vi "svx_Oct_Waterfall Execute.vi"(0 "Data In":T3 {"Plots"."Y" format="%.2f"; "Plots"."X" format="%.2f"}, 1 "Display State In":T2={"X Scale Width %"=80.0, "Y Scale Height %"=40.0, "X-Axis Range"={"Minimum"=0.0, "Maximum"=10.0}, "Y-Axis Range"={"Minimum"=0.0, "Maximum"=10.0}, "Z-Axis Range"={"Minimum"=0.0, "Maximum"=10.0}, "Plot Color"=0, "Frame Color"=61212, "Background Color"=16252785, "Initial AutoScale Y"=TRUE, "AutoScale X"=2, "AutoScale Y"=2, "AutoScale Z"=2, "Plot Transparency"=FALSE, "X-Axis Name"="Frequency", "Y-Axis Name"="Amplitude", "Z-Axis Name"="", "X-Axis Scaling Factor"={"Offset"=0.0, "Multiplier"=1.0}, "Y-Axis Scaling Factor"={"Offset"=0.0, "Multiplier"=1.0}, "Z-Axis Scaling Factor"={"Offset"=0.0, "Multiplier"=1.0}, "X-Scale Visible"=TRUE, "Y-Scale Visible"=TRUE, "Z-Scale Visible"=TRUE, "X-Scale Label Visible"=TRUE, "Y-Scale Label Visible"=TRUE, "Z-Scale Label Visible"=TRUE, "X-Axis Range Scaled"={"Minimum"=0.0, "Maximum"=10.0}, "Y-Axis Range Scaled"={"Minimum"=0.0, "Maximum"=10.0}, "Z-Axis Range Scaled"={"Minimum"=0.0, "Maximum"=10.0}, "Rev Z Order"=FALSE, "X-Scale Format Str"="%#.4g", "Y-Scale Format Str"="%#.4g", "Z-Scale Format Str"="%#.4g", "Decor color"=12369084, "Scale Range Change"=refnum, "out of state queue"=refnum, "property nodes"=refnum} caption="State In", 2 "Container State":T5, 3 "# Plots Updated":i32, 4 "Dec/Cropped in":T3 {"Plots"."Y" format="%.2f"; "Plots"."X" format="%.2f"}, 6 "Execution Tasks":T4[](array[typedef]), 7 "Main Graph":refnum<vi>, 8 "Coords":T1, 9 "XY Scale Graph ref":refnum<vi>, 11 "Z Scale Graph ref":refnum<vi>, 12 "This VI":refnum<vi>, 13 "Background ref":refnum<vi>) -> (14 "Data Out":T3={"z0"=0.0, "dz"=1.0, "Plots"=[]} {"Plots"."Y" format="%.2f"; "Plots"."X" format="%.2f"}, 15 "Display State Out":T2={"X Scale Width %"=80.0, "Y Scale Height %"=40.0, "X-Axis Range"={"Minimum"=0.0, "Maximum"=10.0}, "Y-Axis Range"={"Minimum"=0.0, "Maximum"=10.0}, "Z-Axis Range"={"Minimum"=0.0, "Maximum"=10.0}, "Plot Color"=61212, "Frame Color"=16252785, "Background Color"=16777222, "Initial AutoScale Y"=TRUE, "AutoScale X"=2, "AutoScale Y"=2, "AutoScale Z"=2, "Plot Transparency"=FALSE, "X-Axis Name"="Frequency", "Y-Axis Name"="Amplitude", "Z-Axis Name"="", "X-Axis Scaling Factor"={"Offset"=0.0, "Multiplier"=1.0}, "Y-Axis Scaling Factor"={"Offset"=0.0, "Multiplier"=1.0}, "Z-Axis Scaling Factor"={"Offset"=0.0, "Multiplier"=1.0}, "X-Scale Visible"=TRUE, "Y-Scale Visible"=TRUE, "Z-Scale Visible"=TRUE, "X-Scale Label Visible"=TRUE, "Y-Scale Label Visible"=TRUE, "Z-Scale Label Visible"=TRUE, "X-Axis Range Scaled"={"Minimum"=0.0, "Maximum"=10.0}, "Y-Axis Range Scaled"={"Minimum"=0.0, "Maximum"=10.0}, "Z-Axis Range Scaled"={"Minimum"=0.0, "Maximum"=10.0}, "Rev Z Order"=FALSE, "X-Scale Format Str"="%#.4g", "Y-Scale Format Str"="%#.4g", "Z-Scale Format Str"="%#.4g", "Decor color"=12369084, "Scale Range Change"=refnum, "out of state queue"=refnum, "property nodes"=refnum} caption="State", 17 "# Plots Updated out":i32, 18 "Dec/Cropped out":T3={"z0"=0.0, "dz"=1.0, "Plots"=[]} {"Plots"."Y" format="%.2f"; "Plots"."X" format="%.2f"})   [LabVIEW 2017, in "SVX Octave Waterfall Graph.xctl"]
uses:
  <vilib>/addons/_XControls/Octave Waterfall Graph/SVX Octave Waterfall Graph.xctl
  <vilib>/_xctls/Container State.ctl
  <vilib>/addons/_XControls/Octave Waterfall Graph/subVIs/svx_Oct_Waterfall Data.ctl
  <vilib>/addons/_XControls/Octave Waterfall Graph/subVIs/svx_Oct_Waterfall State.ctl
  <vilib>/addons/_XControls/Octave Waterfall Graph/subVIs/svx_Oct_Waterfall Execution Tasks.ctl
  <vilib>/Utility/miscctls.llb/LVPoint32TypeDef.ctl
  <vilib>/_xctls/XControlSupport.lvlib
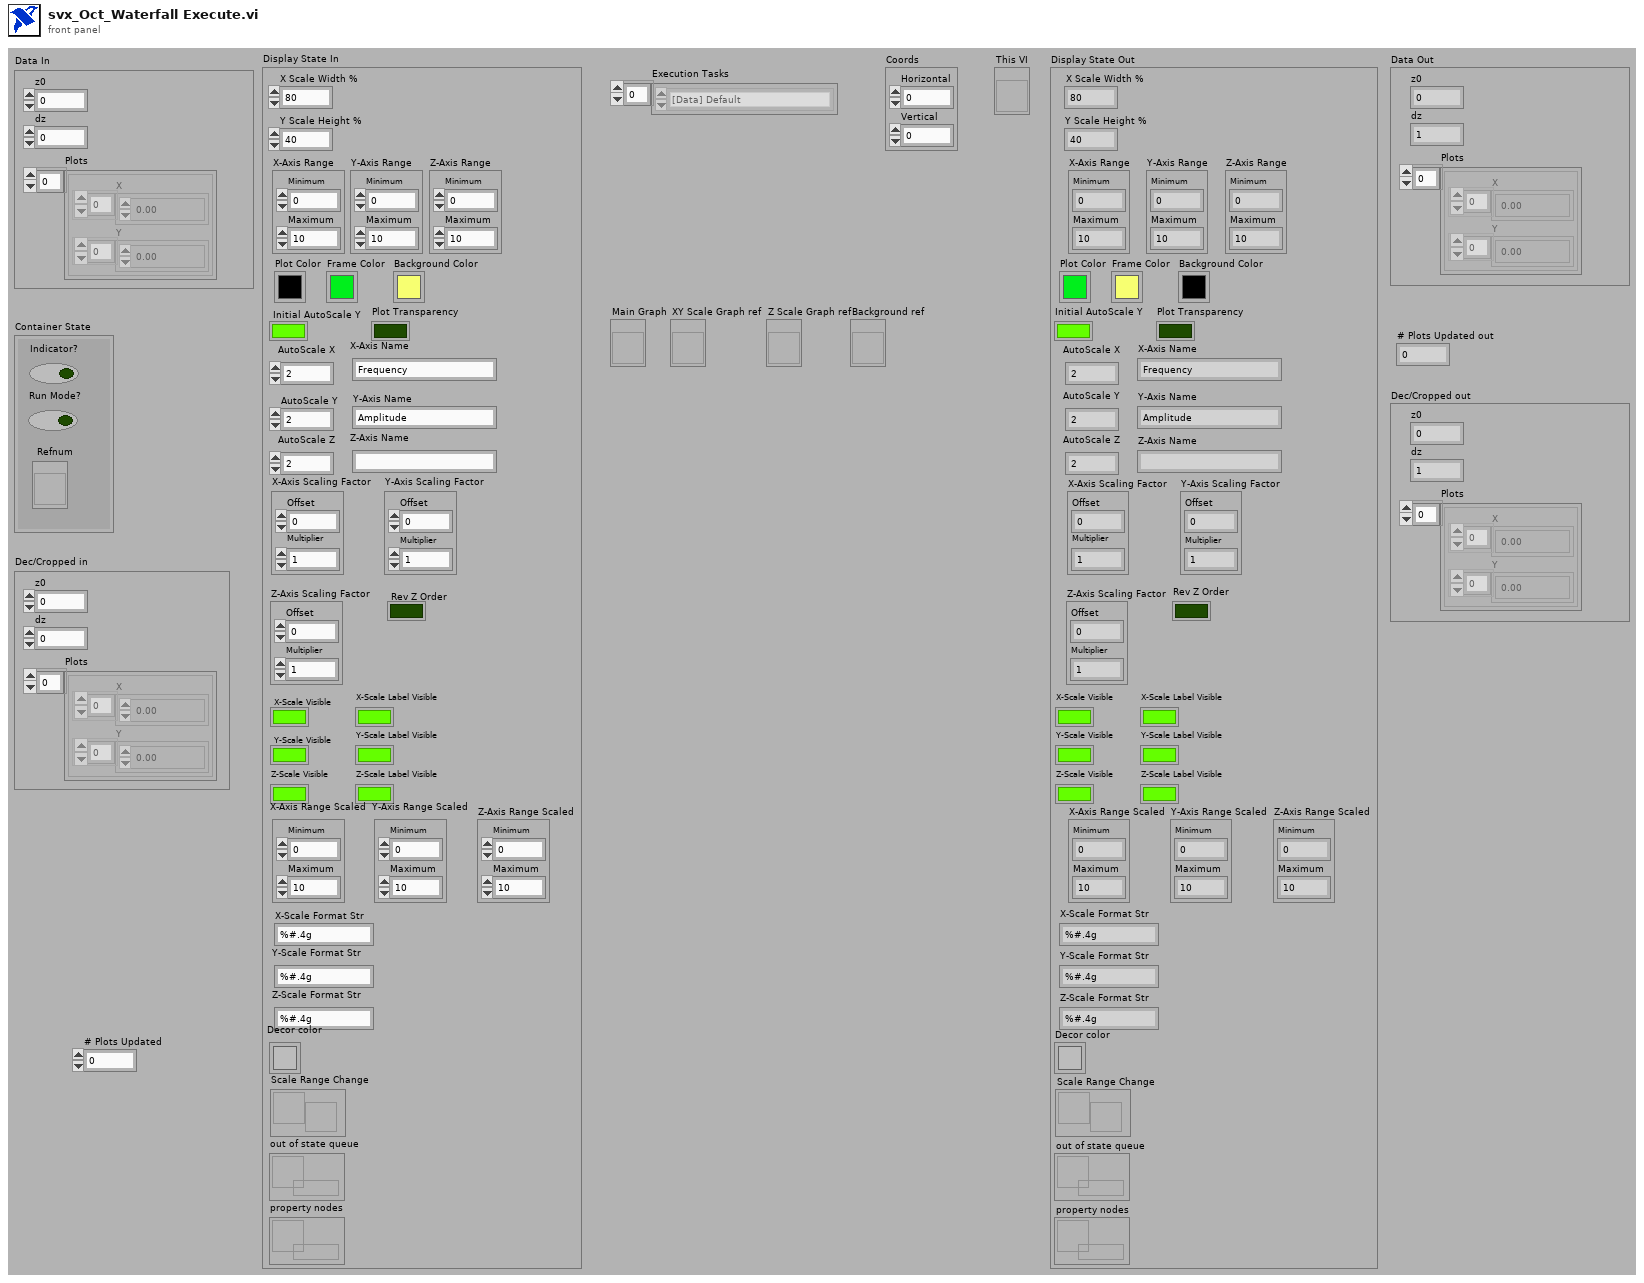
[diagram p1: front panel]
types:
  T1 = typedef "LVPoint32TypeDef.ctl" = cluster{"Horizontal":i32, "Vertical":i32}
  T2 = typedef "SVX Octave Waterfall Graph.xctl/svx_Oct_Waterfall State.ctl" = cluster{"X Scale Width %":dbl, "Y Scale Height %":dbl, "X-Axis Range":cluster{"Minimum":dbl, "Maximum":dbl}, "Y-Axis Range":cluster{"Minimum":dbl, "Maximum":dbl}, "Z-Axis Range":cluster{"Minimum":dbl, "Maximum":dbl}, "Plot Color":u32, "Frame Color":u32, "Background Color":u32, "Initial AutoScale Y":bool, "AutoScale X":u8, "AutoScale Y":u8, "AutoScale Z":u8, "Plot Transparency":bool, "X-Axis Name":string, "Y-Axis Name":string, "Z-Axis Name":string, "X-Axis Scaling Factor":cluster{"Offset":dbl, "Multiplier":dbl}, "Y-Axis Scaling Factor":cluster{"Offset":dbl, "Multiplier":dbl}, "Z-Axis Scaling Factor":cluster{"Offset":dbl, "Multiplier":dbl}, "X-Scale Visible":bool, "Y-Scale Visible":bool, "Z-Scale Visible":bool, "X-Scale Label Visible":bool, "Y-Scale Label Visible":bool, "Z-Scale Label Visible":bool, "X-Axis Range Scaled":cluster{"Minimum":dbl, "Maximum":dbl}, "Y-Axis Range Scaled":cluster{"Minimum":dbl, "Maximum":dbl}, "Z-Axis Range Scaled":cluster{"Minimum":dbl, "Maximum":dbl}, "Rev Z Order":bool, "X-Scale Format Str":string, "Y-Scale Format Str":string, "Z-Scale Format Str":string, "Decor color":u32, "Scale Range Change":refnum<user-event>, "out of state queue":refnum<queue>, "property nodes":refnum<queue>}
  T3 = typedef "SVX Octave Waterfall Graph.xctl/svx_Oct_Waterfall Data.ctl" = cluster{"z0":dbl, "dz":dbl, "Plots":cluster{"X":dbl[], "Y":dbl[]}[]}
  T4 = typedef "SVX Octave Waterfall Graph.xctl/svx_Oct_Waterfall Execution Tasks.ctl" = enum16{"[Data] Default", "[Data] Update Graph", "[Pane] Calculate Size from Coord Change", "[Pane] Calculate Size from Display State", "[Plot] Redraw Frame", "[Plot] Update Plot Color", "[Scale] Autoscale or Crop X, Y, Z", "[Scale] Resize Scales", "[Scale] Align Scale Labels", "[Plot] Initialize Plot", "[Scale] X Scale", "[Scale] Y Scale", "[Scale] Z Scale", "[Scale] Multiplier/Offset", "[Scale] Name", "[Scale] Visible", "[Scale] Label Visible", "[Scale] Format"}
  T5 = typedef "XControlSupport.lvlib/Container State.ctl" = cluster{"Indicator?":bool, "Run Mode?":bool, " Refnum":refnum<vi>}
  T6 = cluster{"Amp Width":u32, "Amp Height":u32, "Z Height":u32, "Wform Height":u32, "Wform Width":u32}
  T7 = cluster{"Width":u16, "Style":enum32{"Solid", "Dash", "Dot", "DashDot", "DashDotDot"}}
  T8 = typedef "LVRectTypeDef.ctl" = cluster{"Left":i16, "Top":i16, "Right":i16, "Bottom":i16}
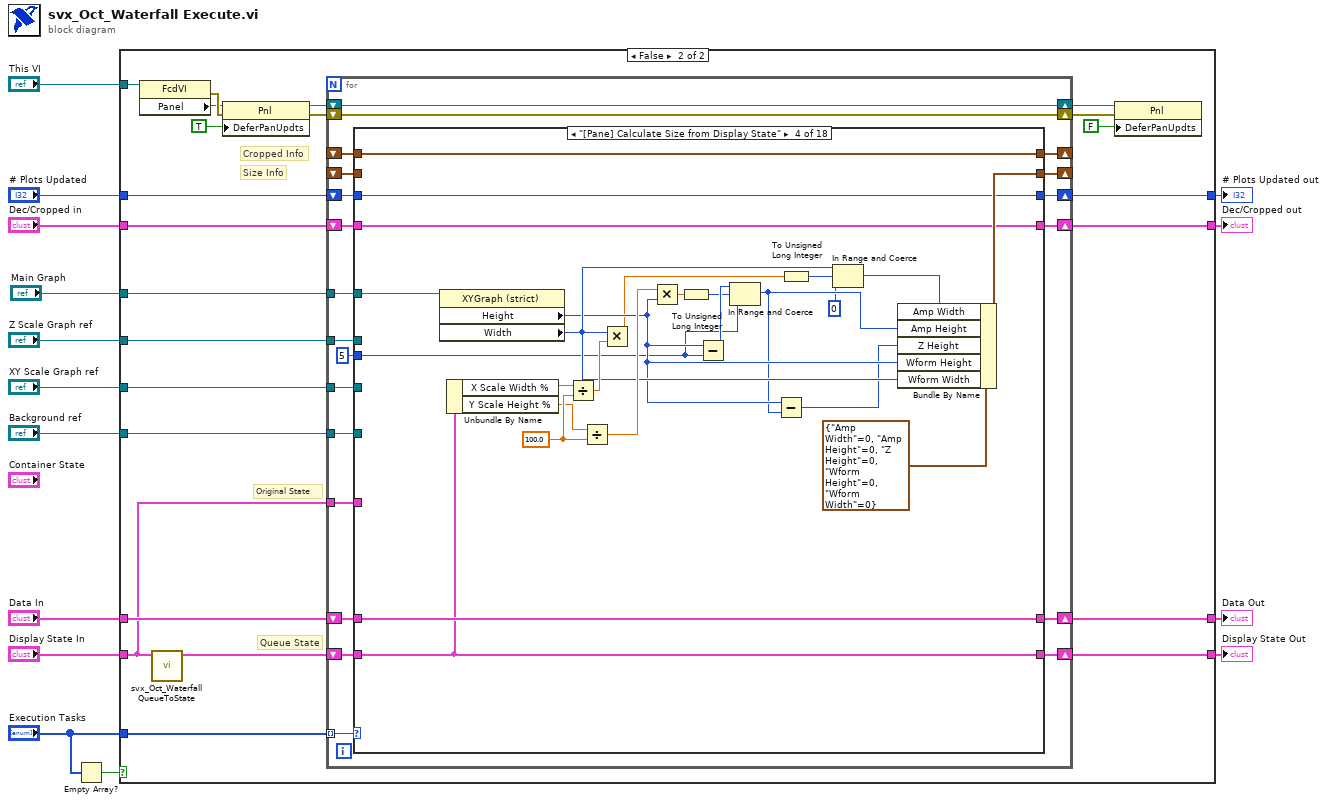
[diagram p0: block diagram]
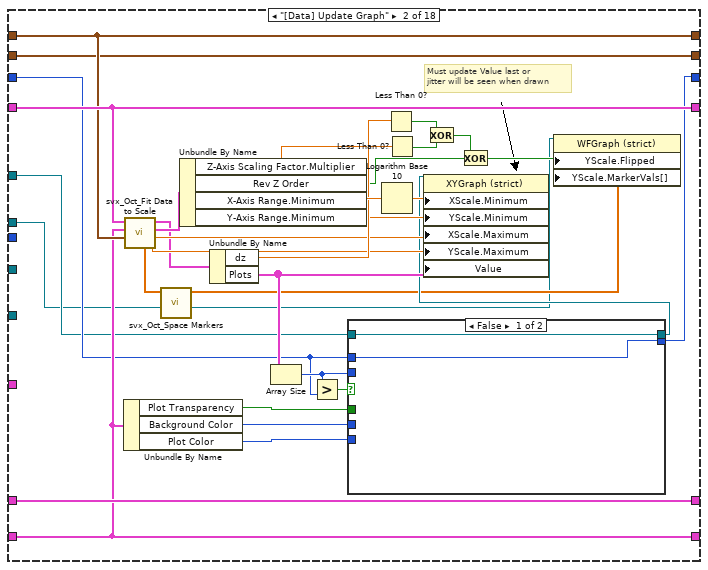
[diagram p4: hidden frame]
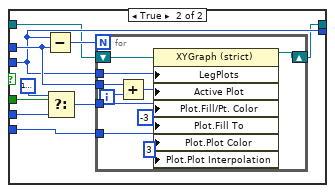
[diagram p5: hidden frame]
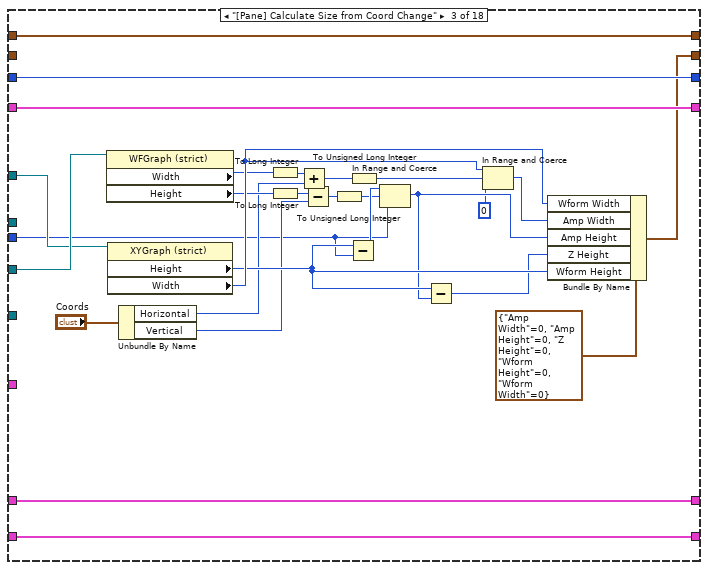
[diagram p6: hidden frame]
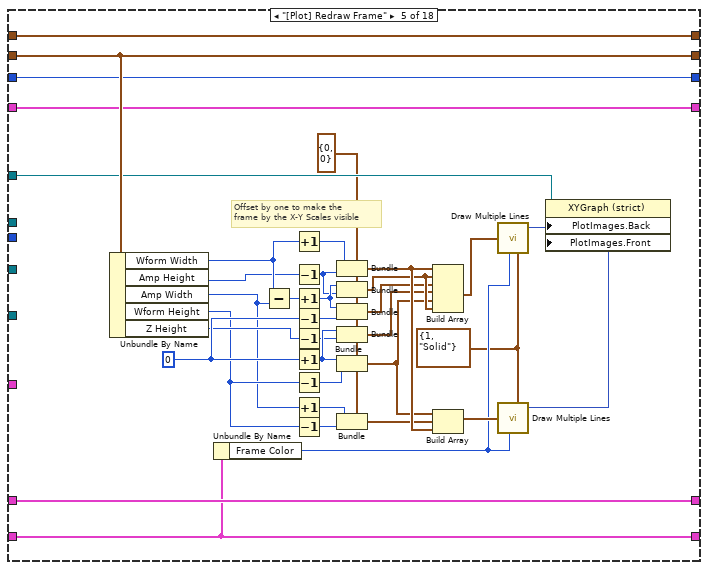
[diagram p7: hidden frame]
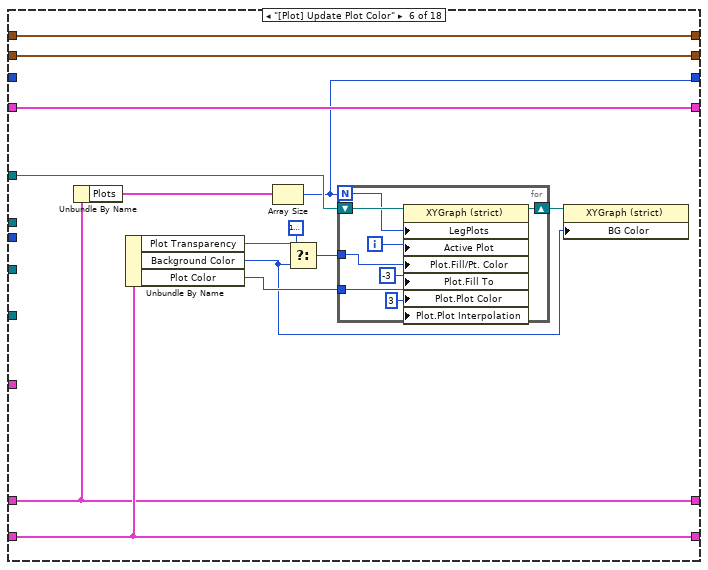
[diagram p8: hidden frame]
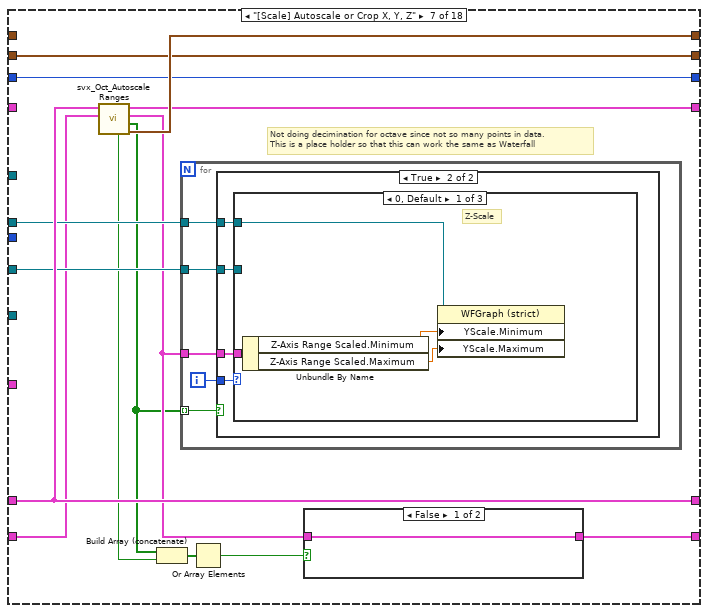
[diagram p9: hidden frame]
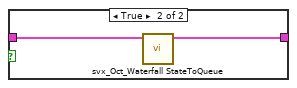
[diagram p10: hidden frame]
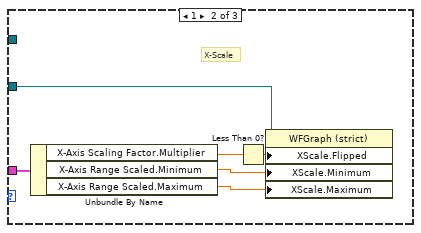
[diagram p12: hidden frame]
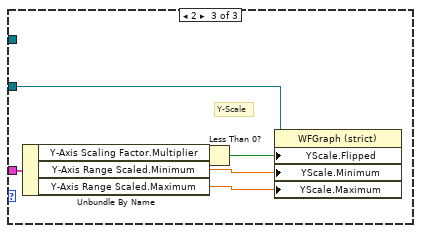
[diagram p13: hidden frame]
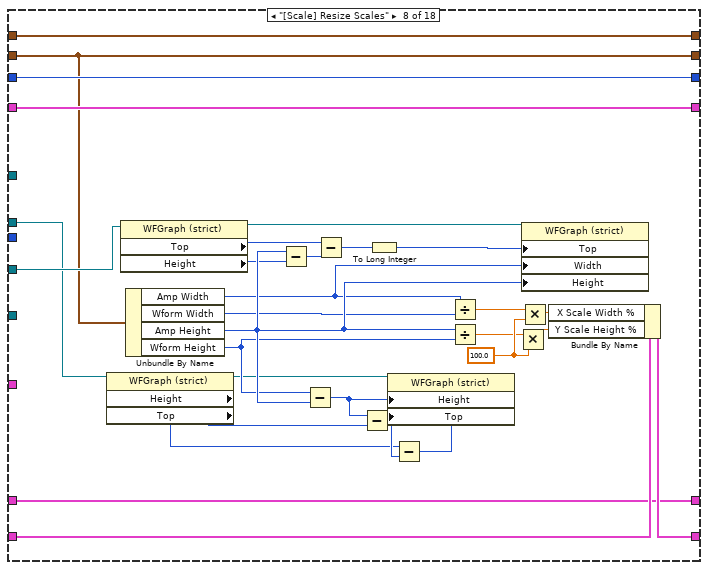
[diagram p14: hidden frame]
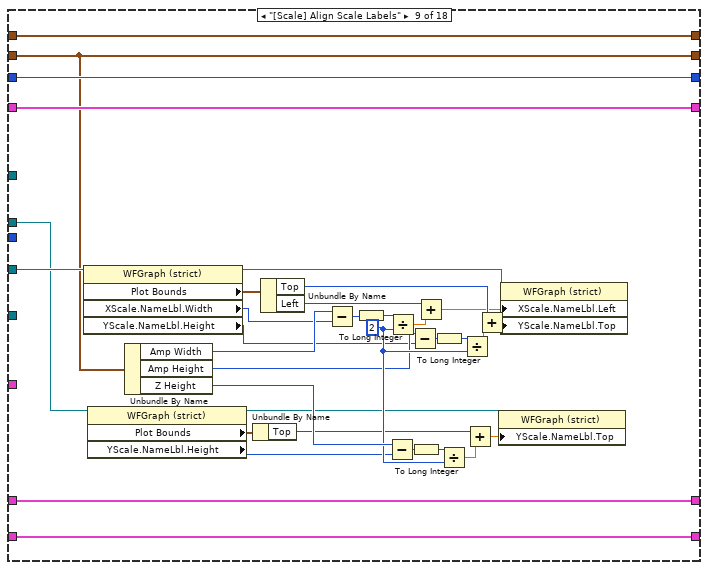
[diagram p15: hidden frame]
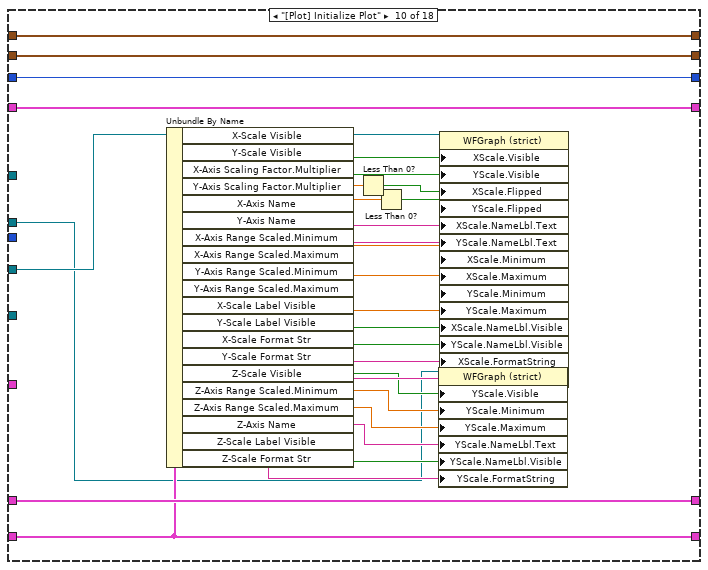
[diagram p16: hidden frame]
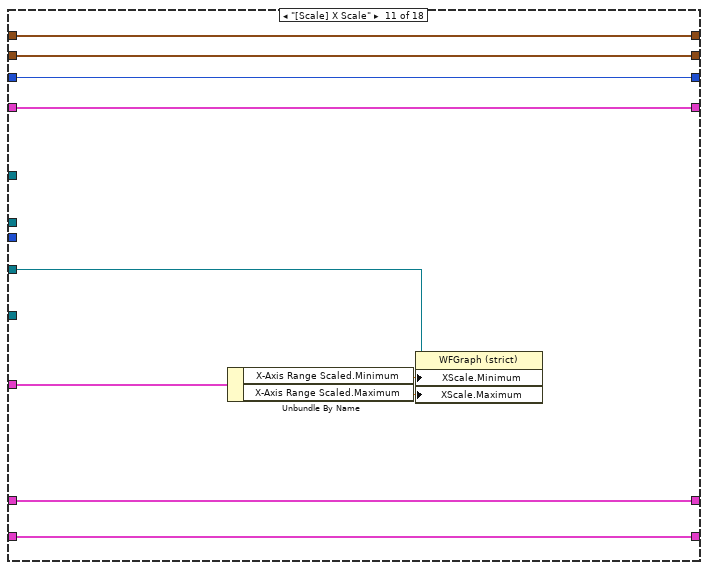
[diagram p17: hidden frame]
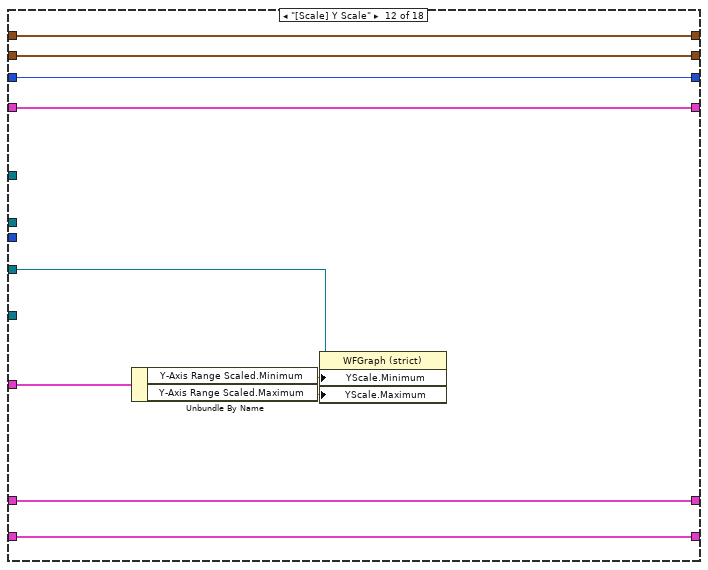
[diagram p18: hidden frame]
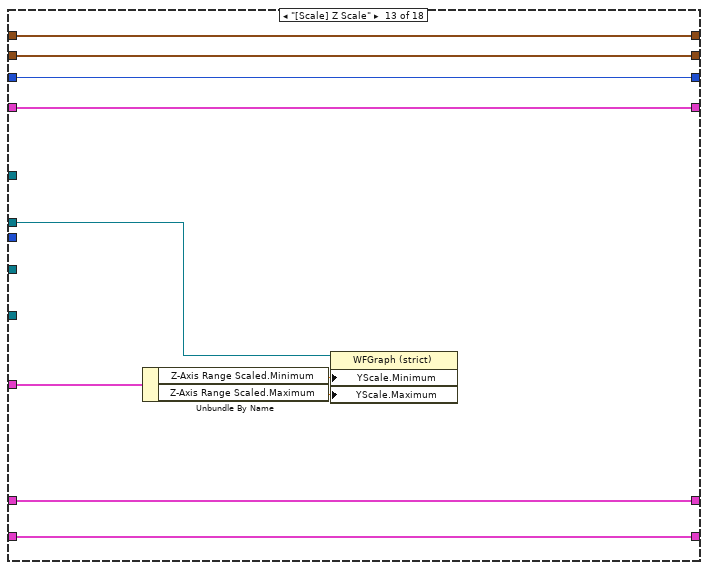
[diagram p19: hidden frame]
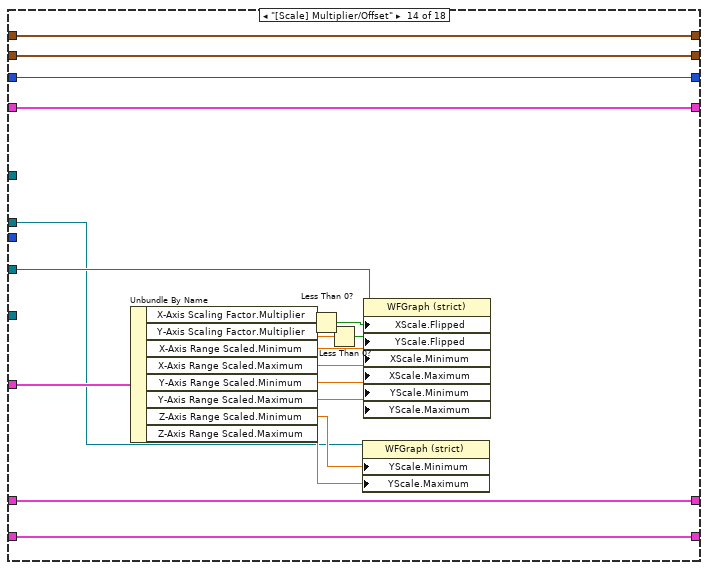
[diagram p20: hidden frame]
diagram:
  n1 = Empty Array?(array="Execution Tasks") -> (empty?=w10:bool)
  n2 = case shown="False" w10 {
    tunnel: "This VI" -> [_ w39]
    tunnel: "Main Graph" -> [_ w23]
    tunnel: "Z Scale Graph ref" -> [_ w22]
    tunnel: "XY Scale Graph ref" -> [_ w21]
    tunnel: "Execution Tasks" -> [_ w33]
    tunnel: "Data In" -> [w18 w28]
    tunnel: [w18 w27] -> w3
    tunnel: [w19 w25] -> w2
    tunnel: "Dec/Cropped in" -> [w17 w30]
    tunnel: [w17 w29] -> w4
    tunnel: "# Plots Updated" -> [w16 w32]
    tunnel: [w16 w31] -> w5
    tunnel: "Background ref" -> [_ w20]
    tunnel: "Display State In" -> [w19 w24]
    frame True {
    }
    frame False {
      # "Cropped Info"
      # "Size Info"
      # "Queue State"
      # "Original State"
      n3 = property class="FcdVI"(reference=w39) -> (error out=w42:errorcluster, "Panel"=w40:refnum<vi>)  [unwired: 1 in, 1 out]
      n4 = call <vilib>:"svx_Oct_Waterfall QueueToState.vi"("State In"=w24) -> ("State Out"=w26:T2)  [unwired: 10 in]
      n5 = property class="Pnl"(reference=w40, error in=w42, "DeferPanUpdts"=TRUE ("Defer Panel Updates")) -> (reference out=w38:refnum<vi>, error out=w35:errorcluster)
      n6 = for {
        shift-right: [w63] -> w36
        shift-left: w38 -> [w63]
        shift-right: [w62] -> w34
        shift-left: w35 -> [w62]
        tunnel: w33 -> [w61] mode=indexing
        shift-right: [w59] -> w31
        shift-left: w32 -> [w60]
        shift-right: [w57] -> w29
        shift-left: w30 -> [w58]
        shift-right: [w56] -> w27
        shift-left: w28 -> [w55]
        shift-right: [w54] -> w25
        shift-left: w26 -> [w53]
        tunnel: w24 -> [w44]
        tunnel: w23 -> [w52]
        tunnel: w22 -> [w51]
        tunnel: w21 -> [w50]
        tunnel: w20 -> [w49]
        shift-right: [w45] -> _
        shift-left: _ -> [w46]
        shift-right: [w47] -> _
        shift-left: _ -> [w48]
        n7 = case shown="\"[Pane] Calculate Size from Display State\"" w61 {
          tunnel: w60 -> [w69 w77 w149 w160 w180 _ w240 w306 w312 w369 w372 w389 w399 w418 w430 w442 w449 w461]
          tunnel: [w69 w76 w149 w160 w180 w216 w240 w306 w312 w369 w372 w389 w399 w418 w430 w442 w449 w461] -> w59
          tunnel: w58 -> [w68 w88 w152 w159 w181 w219 _ w305 w313 w368 w377 w388 w398 w417 w429 w441 w448 w460]
          tunnel: [w68 w88 w152 w159 w181 w219 w247 w305 w313 w368 w377 w388 w398 w417 w429 w441 w448 w460] -> w57
          tunnel: [w67 w87 w150 w164 w184 w224 w248 w279 w309 w367 w374 w387 w397 w416 w428 w440 w453 w465] -> w56
          tunnel: w55 -> [w67 w87 w150 w164 w184 w224 w248 w279 w309 w367 w374 w387 w397 w416 w428 w440 w453 w465]
          tunnel: [w66 w78 w151 w163 w183 w225 w241 w284 w308 w344 w373 w386 w394 w415 w427 w439 w452 w464] -> w54
          tunnel: w53 -> [w66 w78 w151 w163 w183 w225 w242 w285 w308 w344 w373 w386 w394 w415 w427 w439 w452 w464]
          tunnel: w52 -> [_ w75 w130 w162 w182 w222 _ _ _ _ _ _ _ _ _ _ _ _]
          tunnel: w51 -> [_ w71 _ _ _ _ w245 w280 w314 w342 _ _ w393 w402 w421 w433 w445 w457]
          tunnel: w50 -> [_ _ w131 _ _ _ w244 w282 w315 w343 w375 w382 _ w403 w422 w434 w446 w459]
          tunnel: w49 -> [_ _ _ _ _ _ _ _ _ _ _ _ _ _ _ _ _ _]
          tunnel: w48 -> [w65 w86 w132 w158 w179 w214 _ w307 w310 w371 w379 w391 w401 w420 w432 w444 w451 w463]
          tunnel: [w65 w86 w132 w158 w179 w214 w249 w307 w310 w371 w379 w391 w401 w420 w432 w444 w451 w463] -> w47
          tunnel: w46 -> [w64 w85 _ _ w185 w215 w246 w278 w311 w370 w378 w390 w400 w419 w431 w443 w450 w462]
          tunnel: [w64 w85 w133 w161 w185 w215 w246 w278 w311 w370 w378 w390 w400 w419 w431 w443 w450 w462] -> w45
          tunnel: w44 -> [_ _ _ _ _ _ _ _ _ _ w376 w383 w392 w404 w423 w435 w447 w458]
          tunnel: u32 5 ("Plot Area:Size:Height") -> [_ _ w129 w157 _ _ _ _ _ _ _ _ _ _ _ _ _ _]
          frame "[Data] Default", Default {
          }
          frame "[Data] Update Graph" {
            # "Must update Value last or\njitter will be seen when drawn"
            n8 = Unbundle By Name(w78) -> ("Plot Transparency"=w80:bool, "Background Color"=w82:u32, "Plot Color"=w81:u32)
            n9 = call <vilib>:"svx_Oct_Fit Data to Scale.vi"("Cropped Info"=w86, "Display State In"=w78, "Data In"=w88) -> ("Waveform YScale Max"=w92:dbl, "Waveform XScale Max"=w91:dbl, "Display State Out"=w93:T2, "Data Out"=w89:T3, "Markers"=w73:dbl[])  [unwired: 4 in]
            n10 = call <vilib>:"svx_Oct_Space Markers.vi"("Z Scale Graph ref"=w71, "markers in"=w73) -> ("Z Scale Graph ref out"=w70:refnum<vi>, "markers out"=w72:dbl[])  [unwired: 8 in]
            n11 = Unbundle By Name(w93) -> ("Z-Axis Scaling Factor.Multiplier"=w97:dbl, "Rev Z Order"=w98:bool, "X-Axis Range.Minimum"=w101:dbl, "Y-Axis Range.Minimum"=w90:dbl)
            n12 = Unbundle By Name(w89) -> ("dz"=w100:dbl, "Plots"=w79:cluster{"X":dbl[], "Y":dbl[]}[])
            n13 = Array Size(array=w79) -> (size(s)=w83:i32)
            n14 = Greater?(x=w83, y=w77) -> (0:w84:bool)
            n15 = case shown="False" w84 {
              tunnel: w83 -> [_ w107]
              tunnel: w82 -> [_ w109]
              tunnel: w81 -> [_ w114]
              tunnel: w77 -> [w104 w112]
              tunnel: w80 -> [_ w110]
              tunnel: [w104 w107] -> w76
              tunnel: w75 -> [w103 w106]
              tunnel: [w103 w105] -> w74
              frame False {
              }
              frame True {
                n16 = Subtract(x=w107, y=w112) -> (x-y=w113:i32)
                n17 = Select(t=u32 16777216, s=w110, f=w109) -> (s? t:f=w108:u32)
                n18 = for {
                  N: w113 -> [_]
                  tunnel: w114 -> [w124]
                  tunnel: w107 -> [w123]
                  tunnel: w112 -> [w122]
                  tunnel: w108 -> [w118]
                  shift-right: [w115] -> w105
                  shift-left: w106 -> [w116]
                  i -> [w121]
                  n19 = Add(x=w122, y=w121) -> (x+y=w120:i32)
                  n20 = property on="Property Node" class="XYGraph (strict)"(reference=w116, "LegPlots"=w123, "Active Plot"=w120, "Plot.Fill/Pt. Color"=w118, "Plot.Fill To"=i16 -3, "Plot.Plot Color"=w124, "Plot.Plot Interpolation"=u8 3) -> (reference out=w115:refnum<vi>)  [unwired: 1 in, 1 out]
                }
              }
            }
            n21 = Logarithm Base 10(1:w101) -> (0:w102:dbl)
            n22 = Less Than 0?(x=w100) -> (x < 0?=w96:bool)
            n23 = Less Than 0?(x=w97) -> (x < 0?=w95:bool)
            n24 = property on="Property Node" class="XYGraph (strict)"(reference=w74, "XScale.Minimum"=w102, "YScale.Minimum"=w90, "XScale.Maximum"=w91, "YScale.Maximum"=w92, "Value"=w79) -> ()  [unwired: 1 in, 2 out]
            n25 = Exclusive Or(1:w95, 2:w96) -> (0:w94:bool)
            n26 = Exclusive Or(1:w98, 2:w94) -> (0:w99:bool)
            n27 = property on="Property Node" class="WFGraph (strict)"(reference=w70, "YScale.Flipped"=w99, "YScale.MarkerVals[]"=w72) -> ()  [unwired: 1 in, 2 out]
          }
          frame "[Pane] Calculate Size from Coord Change" {
            n28 = property on="Property Node" class="WFGraph (strict)"(reference=w131) -> ("Width"=w141:u32, "Height"=w137:u32)  [unwired: 1 in, 2 out]
            n29 = property on="Property Node" class="XYGraph (strict)"(reference=w130) -> ("Height"=w147:u32, "Width"=w148:u32)  [unwired: 1 in, 2 out]
            n30 = Unbundle By Name("Coords") -> ("Horizontal"=w135:i32, "Vertical"=w138:i32)
            n31 = To Long Integer(number=w141) -> (32bit integer=w140:i32)
            n32 = To Long Integer(number=w137) -> (32bit integer=w139:i32)
            n33 = Add(x=w140, y=w135) -> (x+y=w126:i32)
            n34 = Subtract(x=w139, y=w138) -> (x-y=w128:i32)
            n35 = To Unsigned Long Integer(number=w128) -> (unsigned 32bit integer=w127:u32)
            n36 = Subtract(x=w147, y=w129) -> (x-y=w136:u32)
            n37 = To Unsigned Long Integer(number=w126) -> (unsigned 32bit integer=w125:u32)
            n38 = In Range and Coerce(upper limit=w136, x=w127, lower limit=w129) -> (coerced(x)=w144:u32)  [unwired: 1 out]
            n39 = Subtract(x=w147, y=w144) -> (x-y=w145:u32)
            n40 = In Range and Coerce(upper limit=w148, x=w125, lower limit=u32 0) -> (coerced(x)=w143:u32)  [unwired: 1 out]
            n41 = Bundle By Name(cluster=T6 {"Amp Width"=0, "Amp Height"=0, "Z Height"=0, "Wform Height"=0, "Wform Width"=0}, "Wform Width"=w148, "Amp Width"=w143, "Amp Height"=w144, "Z Height"=w145, "Wform Height"=w147) -> (w133:T6)
          }
          frame "[Pane] Calculate Size from Display State" {
            w177 = 100.0 ("y")
            n42 = property on="Property Node" class="XYGraph (strict)"(reference=w162) -> ("Height"=w171:u32, "Width"=w172:u32)  [unwired: 1 in, 2 out]
            n43 = Unbundle By Name(w163) -> ("X Scale Width %"=w175:dbl, "Y Scale Height %"=w173:dbl)
            n44 = Divide(x=w175, y=w177) -> (x/y=w176:dbl)
            n45 = Divide(x=w173, y=w177) -> (x/y=w174:dbl)
            n46 = Multiply(x=w172, y=w176) -> (x*y=w156:dbl)
            n47 = Multiply(x=w174, y=w171) -> (x*y=w154:dbl)
            n48 = To Unsigned Long Integer(number=w154) -> (unsigned 32bit integer=w153:u32)
            n49 = Subtract(x=w171, y=w157) -> (x-y=w165:u32)
            n50 = In Range and Coerce(upper limit=w165, x=w153, lower limit=w157) -> (coerced(x)=w169:u32)  [unwired: 1 out]
            n51 = Subtract(x=w171, y=w169) -> (x-y=w170:u32)
            n52 = To Unsigned Long Integer(number=w156) -> (unsigned 32bit integer=w155:u32)
            n53 = In Range and Coerce(upper limit=w172, x=w155, lower limit=u32 0) -> (coerced(x)=w168:u32)  [unwired: 1 out]
            n54 = Bundle By Name(cluster=T6 {"Amp Width"=0, "Amp Height"=0, "Z Height"=0, "Wform Height"=0, "Wform Width"=0}, "Amp Width"=w168, "Amp Height"=w169, "Z Height"=w170, "Wform Height"=w171, "Wform Width"=w172) -> (w161:T6)
          }
          frame "[Plot] Redraw Frame" {
            w178 = cluster{"x":i16, "y":i16} {"x"=0, "y"=0} ("cluster")
            w187 = T7 {"Width"=1, "Style"=enum."Solid"} ("pen")
            w210 = u32 0 ("Offset")
            # "Offset by one to make the\nframe by the X-Y Scales visible"
            n55 = Unbundle By Name(w185) -> ("Wform Width"=w203:u32, "Amp Height"=w201:u32, "Amp Width"=w197:u32, "Wform Height"=w199:u32, "Z Height"=w208:u32)
            n56 = Unbundle By Name(w183) -> ("Frame Color"=w189:u32)
            n57 = Subtract(x=w203, y=w197) -> (x-y=w205:u32)
            n58 = Increment(x=w203) -> (x+1=w204:u32)
            n59 = Decrement(x=w201) -> (x-1=w202:u32)
            n60 = Increment(x=w205) -> (x+1=w206:u32)
            n61 = Decrement(x=w210) -> (x-1=w209:u32)
            n62 = Decrement(x=w208) -> (x-1=w207:u32)
            n63 = Increment(x=w210) -> (x+1=w211:u32)
            n64 = Decrement(x=w199) -> (x-1=w196:u32)
            n65 = Increment(x=w197) -> (x+1=w198:u32)
            n66 = Decrement(x=w199) -> (x-1=w200:u32)
            n67 = Bundle(cluster=w178, "x"=w204, "y"=w202) -> (w195:cluster{"x":i16, "y":i16})
            n68 = Bundle(cluster=w178, "x"=w206, "y"=w202) -> (w194:cluster{"x":i16, "y":i16})
            n69 = Bundle(cluster=w178, "x"=w206, "y"=w209) -> (w190:cluster{"x":i16, "y":i16})
            n70 = Bundle(cluster=w178, "x"=w211, "y"=w207) -> (w191:cluster{"x":i16, "y":i16})
            n71 = Bundle(cluster=w178, "x"=w211, "y"=w196) -> (w193:cluster{"x":i16, "y":i16})
            n72 = Bundle(cluster=w178, "x"=w198, "y"=w200) -> (w192:cluster{"x":i16, "y":i16})
            n73 = Build Array(w195, w194, w190, w191, w193, w194) -> (w212:cluster{"x":i16, "y":i16}[])
            n74 = Build Array(w193, w192, w195) -> (w213:cluster{"x":i16, "y":i16}[])
            n75 = call <vilib>:"Draw Multiple Lines.vi"("line endpoints"=w212, "color(black)"=w189, "pen"=w187) -> ("new picture"=w186:picture)  [unwired: 6 in]
            n76 = call <vilib>:"Draw Multiple Lines.vi"("line endpoints"=w213, "color(black)"=w189, "pen"=w187) -> ("new picture"=w188:picture)  [unwired: 6 in]
            n77 = property on="Property Node" class="XYGraph (strict)"(reference=w182, "PlotImages.Back"=w186, "PlotImages.Front"=w188) -> ()  [unwired: 1 in, 2 out]
          }
          frame "[Plot] Update Plot Color" {
            n78 = Unbundle By Name(w224) -> ("Plots"=w223:cluster{"X":dbl[], "Y":dbl[]}[])
            n79 = Unbundle By Name(w225) -> ("Plot Transparency"=w226:bool, "Background Color"=w217:u32, "Plot Color"=w227:u32)
            n80 = Array Size(array=w223) -> (size(s)=w216:i32)
            n81 = Select(t=u32 16777216, s=w226, f=w217) -> (s? t:f=w220:u32)
            n82 = for {
              N: w216 -> [w229]
              tunnel: w227 -> [w235]
              tunnel: w220 -> [w233]
              shift-right: [w230] -> w218
              shift-left: w222 -> [w231]
              i -> [w228]
              n83 = property on="Property Node" class="XYGraph (strict)"(reference=w231, "LegPlots"=w229, "Active Plot"=w228, "Plot.Fill/Pt. Color"=w233, "Plot.Fill To"=i16 -3, "Plot.Plot Color"=w235, "Plot.Plot Interpolation"=u8 3) -> (reference out=w230:refnum<vi>)  [unwired: 1 in, 1 out]
            }
            n84 = property on="Property Node" class="XYGraph (strict)"(reference=w218, "BG Color"=w217) -> ()  [unwired: 1 in, 2 out]
          }
          frame "[Scale] Autoscale or Crop X, Y, Z" {
            # "Not doing decimination for octave since not so many points in data.\nThis is a place holder so that this can work the same as Waterfall"
            n85 = call <vilib>:"svx_Oct_Autoscale Ranges.vi"("Display State In"=w242, "Data Array In"=w248) -> ("Cropped Info out"=w249:cluster{"First Index":i32, "Length":i32}, "Update Ranges"=w238:bool[], "Display State Out"=w239:T2, "Data Array Out"=w247:T3, "Update Autoscale"=w236:bool)  [unwired: 5 in]
            n86 = Build Array (concatenate)(w238, w236) -> (w237:bool[])
            n87 = for {
              tunnel: w238 -> [w257] mode=indexing
              tunnel: w239 -> [w255]
              tunnel: w245 -> [w254]
              tunnel: w244 -> [w253]
              i -> [w256]
              n88 = case shown="True" w257 {
                tunnel: w256 -> [_ w261]
                tunnel: w255 -> [_ w260]
                tunnel: w254 -> [_ w259]
                tunnel: w253 -> [_ w258]
                frame False {
                }
                frame True {
                  n89 = case shown="0, Default" w261 {
                    tunnel: w260 -> [w265 w271 w277]
                    tunnel: w259 -> [w262 _ _]
                    tunnel: w258 -> [_ w266 w272]
                    frame 0, Default {
                      # "Z-Scale"
                      n90 = Unbundle By Name(w265) -> ("Z-Axis Range Scaled.Minimum"=w264:dbl, "Z-Axis Range Scaled.Maximum"=w263:dbl)
                      n91 = property on="Property Node" class="WFGraph (strict)"(reference=w262, "YScale.Minimum"=w264, "YScale.Maximum"=w263) -> ()  [unwired: 1 in, 2 out]
                    }
                    frame 1 {
                      # "X-Scale"
                      n92 = Unbundle By Name(w271) -> ("X-Axis Scaling Factor.Multiplier"=w270:dbl, "X-Axis Range Scaled.Minimum"=w268:dbl, "X-Axis Range Scaled.Maximum"=w267:dbl)
                      n93 = Less Than 0?(x=w270) -> (x < 0?=w269:bool)
                      n94 = property on="Property Node" class="WFGraph (strict)"(reference=w266, "XScale.Flipped"=w269, "XScale.Minimum"=w268, "XScale.Maximum"=w267) -> ()  [unwired: 1 in, 2 out]
                    }
                    frame 2 {
                      # "Y-Scale"
                      n95 = Unbundle By Name(w277) -> ("Y-Axis Scaling Factor.Multiplier"=w276:dbl, "Y-Axis Range Scaled.Minimum"=w274:dbl, "Y-Axis Range Scaled.Maximum"=w273:dbl)
                      n96 = Less Than 0?(x=w276) -> (x < 0?=w275:bool)
                      n97 = property on="Property Node" class="WFGraph (strict)"(reference=w272, "YScale.Flipped"=w275, "YScale.Minimum"=w274, "YScale.Maximum"=w273) -> ()  [unwired: 1 in, 2 out]
                    }
                  }
                }
              }
            }
            n98 = Or Array Elements(Boolean array=w237) -> (logical OR=w243:bool)
            n99 = case shown="False" w243 {
              tunnel: w239 -> [w250 w252]
              tunnel: [w250 w251] -> w241
              frame False {
              }
              frame True {
                n100 = call <vilib>:"svx_Oct_Waterfall StateToQueue.vi"("State In"=w252) -> ("State Out"=w251:T2)  [unwired: 10 in]
              }
            }
          }
          frame "[Scale] Resize Scales" {
            w298 = 100.0 ("x/y")
            n101 = property on="Property Node" class="WFGraph (strict)"(reference=w280) -> (reference out=w281:refnum<vi>, "Height"=w286:u32, "Top"=w287:i32)  [unwired: 1 in, 1 out]
            n102 = property on="Property Node" class="WFGraph (strict)"(reference=w282) -> (reference out=w283:refnum<vi>, "Top"=w290:i32, "Height"=w293:u32)  [unwired: 1 in, 1 out]
            n103 = Unbundle By Name(w278) -> ("Amp Width"=w301:u32, "Wform Width"=w295:u32, "Amp Height"=w302:u32, "Wform Height"=w294:u32)
            n104 = Subtract(x=w302, y=w293) -> (x-y=w291:u32)
            n105 = Subtract(x=w294, y=w302) -> (x-y=w292:u32)
            n106 = Subtract(x=w290, y=w291) -> (x-y=w303:u32)
            n107 = Subtract(x=w292, y=w286) -> (x-y=w288:u32)
            n108 = To Long Integer(number=w303) -> (32bit integer=w304:i32)
            n109 = Subtract(x=w287, y=w288) -> (x-y=w289:u32)
            n110 = property on="Property Node" class="WFGraph (strict)"(reference=w281, "Height"=w292, "Top"=w289) -> ()  [unwired: 1 in, 2 out]
            n111 = Divide(x=w301, y=w295) -> (x/y=w297:dbl)
            n112 = Divide(x=w302, y=w294) -> (x/y=w296:dbl)
            n113 = Multiply(x=w296, y=w298) -> (x*y=w299:dbl)
            n114 = Multiply(x=w297, y=w298) -> (x*y=w300:dbl)
            n115 = property on="Property Node" class="WFGraph (strict)"(reference=w283, "Top"=w304, "Width"=w301, "Height"=w302) -> ()  [unwired: 1 in, 2 out]
            n116 = Bundle By Name(cluster=w285, "X Scale Width %"=w300, "Y Scale Height %"=w299) -> (w284:T2)
          }
          frame "[Scale] Align Scale Labels" {
            w340 = u32 2 ("y")
            n117 = property on="Property Node" class="WFGraph (strict)"(reference=w315) -> (reference out=w316:refnum<vi>, "Plot Bounds"=w326:T8, "XScale.NameLbl.Width"=w319:u32, "YScale.NameLbl.Height"=w323:u32)  [unwired: 1 in, 1 out]
            n118 = property on="Property Node" class="WFGraph (strict)"(reference=w314) -> (reference out=w317:refnum<vi>, "Plot Bounds"=w337:T8, "YScale.NameLbl.Height"=w334:u32)  [unwired: 1 in, 1 out]
            n119 = Unbundle By Name(w311) -> ("Amp Width"=w331:u32, "Amp Height"=w332:u32, "Z Height"=w341:u32)
            n120 = Unbundle By Name(w337) -> ("Top"=w335:i16)
            n121 = Unbundle By Name(w326) -> ("Top"=w327:i16, "Left"=w325:i16)
            n122 = Subtract(x=w331, y=w319) -> (x-y=w329:u32)
            n123 = To Long Integer(number=w329) -> (32bit integer=w330:i32)
            n124 = Subtract(x=w341, y=w334) -> (x-y=w338:u32)
            n125 = Divide(x=w330, y=w340) -> (x/y=w318:dbl)
            n126 = Subtract(x=w332, y=w323) -> (x-y=w322:u32)
            n127 = To Long Integer(number=w338) -> (32bit integer=w339:i32)
            n128 = Add(x=w325, y=w318) -> (x+y=w320:dbl)
            n129 = To Long Integer(number=w322) -> (32bit integer=w328:i32)
            n130 = Divide(x=w339, y=w340) -> (x/y=w336:dbl)
            n131 = Divide(x=w328, y=w340) -> (x/y=w321:dbl)
            n132 = Add(x=w335, y=w336) -> (x+y=w333:dbl)
            n133 = Add(x=w327, y=w321) -> (x+y=w324:dbl)
            n134 = property on="Property Node" class="WFGraph (strict)"(reference=w317, "YScale.NameLbl.Top"=w333) -> ()  [unwired: 1 in, 2 out]
            n135 = property on="Property Node" class="WFGraph (strict)"(reference=w316, "XScale.NameLbl.Left"=w320, "YScale.NameLbl.Top"=w324) -> ()  [unwired: 1 in, 2 out]
          }
          frame "[Plot] Initialize Plot" {
            n136 = Unbundle By Name(w344) -> ("X-Scale Visible"=w359:bool, "Y-Scale Visible"=w358:bool, "X-Axis Scaling Factor.Multiplier"=w356:dbl, "Y-Axis Scaling Factor.Multiplier"=w355:dbl, "X-Axis Name"=w347:string, "Y-Axis Name"=w348:string, "X-Axis Range Scaled.Minimum"=w349:dbl, "X-Axis Range Scaled.Maximum"=w350:dbl, "Y-Axis Range Scaled.Minimum"=w351:dbl, "Y-Axis Range Scaled.Maximum"=w352:dbl, "X-Scale Label Visible"=w363:bool, "Y-Scale Label Visible"=w362:bool, "X-Scale Format Str"=w364:string, "Y-Scale Format Str"=w365:string, "Z-Scale Visible"=w360:bool, "Z-Axis Range Scaled.Minimum"=w353:dbl, "Z-Axis Range Scaled.Maximum"=w354:dbl, "Z-Axis Name"=w357:string, "Z-Scale Label Visible"=w361:bool, "Z-Scale Format Str"=w366:string)
            n137 = Less Than 0?(x=w356) -> (x < 0?=w345:bool)
            n138 = Less Than 0?(x=w355) -> (x < 0?=w346:bool)
            n139 = property on="Property Node" class="WFGraph (strict)"(reference=w342, "YScale.Visible"=w360, "YScale.Minimum"=w353, "YScale.Maximum"=w354, "YScale.NameLbl.Text"=w357, "YScale.NameLbl.Visible"=w361, "YScale.FormatString"=w366) -> ()  [unwired: 1 in, 2 out]
            n140 = property on="Property Node" class="WFGraph (strict)"(reference=w343, "XScale.Visible"=w359, "YScale.Visible"=w358, "XScale.Flipped"=w345, "YScale.Flipped"=w346, "XScale.NameLbl.Text"=w347, "YScale.NameLbl.Text"=w348, "XScale.Minimum"=w349, "XScale.Maximum"=w350, "YScale.Minimum"=w351, "YScale.Maximum"=w352, "XScale.NameLbl.Visible"=w363, "YScale.NameLbl.Visible"=w362, "XScale.FormatString"=w364, "YScale.FormatString"=w365) -> ()  [unwired: 1 in, 2 out]
          }
          frame "[Scale] X Scale" {
            n141 = Unbundle By Name(w376) -> ("X-Axis Range Scaled.Minimum"=w380:dbl, "X-Axis Range Scaled.Maximum"=w381:dbl)
            n142 = property on="Property Node" class="WFGraph (strict)"(reference=w375, "XScale.Minimum"=w380, "XScale.Maximum"=w381) -> ()  [unwired: 1 in, 2 out]
          }
          frame "[Scale] Y Scale" {
            n143 = Unbundle By Name(w383) -> ("Y-Axis Range Scaled.Minimum"=w384:dbl, "Y-Axis Range Scaled.Maximum"=w385:dbl)
            n144 = property on="Property Node" class="WFGraph (strict)"(reference=w382, "YScale.Minimum"=w384, "YScale.Maximum"=w385) -> ()  [unwired: 1 in, 2 out]
          }
          frame "[Scale] Z Scale" {
            n145 = Unbundle By Name(w392) -> ("Z-Axis Range Scaled.Minimum"=w395:dbl, "Z-Axis Range Scaled.Maximum"=w396:dbl)
            n146 = property on="Property Node" class="WFGraph (strict)"(reference=w393, "YScale.Minimum"=w395, "YScale.Maximum"=w396) -> ()  [unwired: 1 in, 2 out]
          }
          frame "[Scale] Multiplier/Offset" {
            n147 = Unbundle By Name(w404) -> ("X-Axis Scaling Factor.Multiplier"=w413:dbl, "Y-Axis Scaling Factor.Multiplier"=w412:dbl, "X-Axis Range Scaled.Minimum"=w407:dbl, "X-Axis Range Scaled.Maximum"=w414:dbl, "Y-Axis Range Scaled.Minimum"=w408:dbl, "Y-Axis Range Scaled.Maximum"=w409:dbl, "Z-Axis Range Scaled.Minimum"=w410:dbl, "Z-Axis Range Scaled.Maximum"=w411:dbl)
            n148 = Less Than 0?(x=w413) -> (x < 0?=w405:bool)
            n149 = Less Than 0?(x=w412) -> (x < 0?=w406:bool)
            n150 = property on="Property Node" class="WFGraph (strict)"(reference=w402, "YScale.Minimum"=w410, "YScale.Maximum"=w411) -> ()  [unwired: 1 in, 2 out]
            n151 = property on="Property Node" class="WFGraph (strict)"(reference=w403, "XScale.Flipped"=w405, "YScale.Flipped"=w406, "XScale.Minimum"=w407, "XScale.Maximum"=w414, "YScale.Minimum"=w408, "YScale.Maximum"=w409) -> ()  [unwired: 1 in, 2 out]
          }
          frame "[Scale] Name" {
            n152 = Unbundle By Name(w423) -> ("X-Axis Name"=w424:string, "Y-Axis Name"=w425:string, "Z-Axis Name"=w426:string)
            n153 = property on="Property Node" class="WFGraph (strict)"(reference=w422, "XScale.NameLbl.Text"=w424, "YScale.NameLbl.Text"=w425) -> ()  [unwired: 1 in, 2 out]
            n154 = property on="Property Node" class="WFGraph (strict)"(reference=w421, "YScale.NameLbl.Text"=w426) -> ()  [unwired: 1 in, 2 out]
          }
          frame "[Scale] Visible" {
            n155 = Unbundle By Name(w435) -> ("X-Scale Visible"=w436:bool, "Y-Scale Visible"=w437:bool, "Z-Scale Visible"=w438:bool)
            n156 = property on="Property Node" class="WFGraph (strict)"(reference=w434, "XScale.Visible"=w436, "YScale.Visible"=w437) -> ()  [unwired: 1 in, 2 out]
            n157 = property on="Property Node" class="WFGraph (strict)"(reference=w433, "YScale.Visible"=w438) -> ()  [unwired: 1 in, 2 out]
          }
          frame "[Scale] Label Visible" {
            n158 = Unbundle By Name(w447) -> ("X-Scale Label Visible"=w454:bool, "Y-Scale Label Visible"=w455:bool, "Z-Scale Label Visible"=w456:bool)
            n159 = property on="Property Node" class="WFGraph (strict)"(reference=w446, "XScale.NameLbl.Visible"=w454, "YScale.NameLbl.Visible"=w455) -> ()  [unwired: 1 in, 2 out]
            n160 = property on="Property Node" class="WFGraph (strict)"(reference=w445, "YScale.NameLbl.Visible"=w456) -> ()  [unwired: 1 in, 2 out]
          }
          frame "[Scale] Format" {
            n161 = Unbundle By Name(w458) -> ("X-Scale Format Str"=w466:string, "Y-Scale Format Str"=w467:string, "Z-Scale Format Str"=w468:string)
            n162 = property on="Property Node" class="WFGraph (strict)"(reference=w459, "XScale.FormatString"=w466, "YScale.FormatString"=w467) -> ()  [unwired: 1 in, 2 out]
            n163 = property on="Property Node" class="WFGraph (strict)"(reference=w457, "YScale.FormatString"=w468) -> ()  [unwired: 1 in, 2 out]
          }
        }
      }
      n164 = property class="Pnl"(reference=w36, error in=w34, "DeferPanUpdts"=FALSE ("Defer Panel Updates")) -> ()  [unwired: 2 out]
    }
  }
  "# Plots Updated out" <- w5
  "Dec/Cropped out" <- w4
  "Data Out" <- w3
  "Display State Out" <- w2
